vi "Set Print.vi"(8 "error in (no error)":errorcluster, 10 "On?":bool, 11 "MFC in":refnum<class "MFC.lvclass">) -> (0 "error out":errorcluster, 3 "MFC out":refnum<class "MFC.lvclass">)   [LabVIEW 2018, in "MFC Actor.lvlib" / "MFC.lvclass"]
uses:
  MFC.lvclass
  C:/Program Files/National Instruments/LabVIEW 2018/vi.lib/ActorFramework/Actor/Actor.lvclass
  <vilib>/ActorFramework/Actor/Actor.lvclass/Actor.ctl
  <vilib>/ActorFramework/Message Enqueuer/Message Enqueuer.lvclass/Message Enqueuer.ctl
  MFC.lvclass/MFC.ctl
  MFC Messages/Change Setpoint Msg/Change Setpoint Msg.lvclass/Change Setpoint Msg.ctl
  <vilib>/ActorFramework/Message Enqueuer/Init from Existing Queue.vi
  <vilib>/ActorFramework/Message Enqueuer/Enqueue.vi
  MFC Messages/Change Setpoint Msg/Change Setpoint Msg.lvclass
  C:/Program Files/National Instruments/LabVIEW 2018/vi.lib/ActorFramework/Message/Message.lvclass
  <vilib>/ActorFramework/Message Priority Queue/Priority Enqueue.vi
  <vilib>/ActorFramework/Message Enqueuer/Message Enqueuer.lvclass
  <vilib>/ActorFramework/Actor/Actor.lvclass
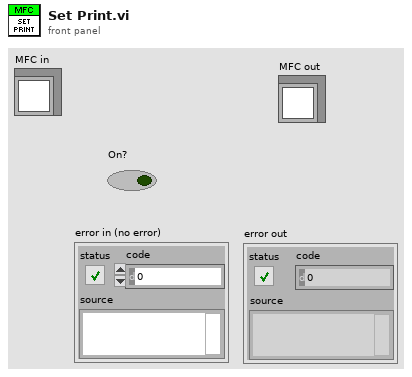
[diagram p1: front panel]
types:
  T1 = enum8{"Enabled", "Disabled", "Disabled and Grayed Out"}
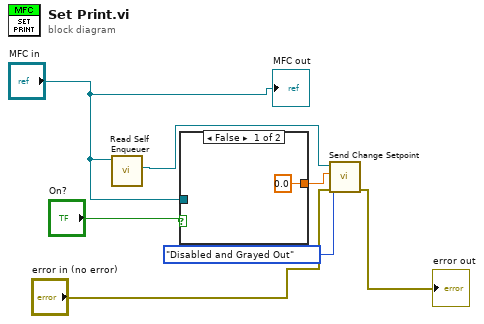
[diagram p0: block diagram]
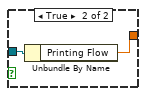
[diagram p2: hidden frame]
diagram:
  n1 = call <vilib>:"Read Self Enqueuer.vi"("Actor"="MFC in") -> ("Self Enqueuer"=w6:refnum<class "Message Enqueuer.lvclass">)  [unwired: 10 in]
  n2 = case shown="False" "On?" {
    tunnel: "MFC in" -> [_ w10]
    tunnel: [0.0 ("Printing Flow") w9] -> w5
    frame False {
    }
    frame True {
      n3 = Unbundle By Name(w10) -> ("Printing Flow"=w9:dbl)
    }
  }
  n4 = call "Send Change Setpoint.vi"("error in (no error)"="error in (no error)", "Disabled"=T1."Disabled and Grayed Out", "Setpoint"=w5, "Message Enqueuer in"=w6) -> ("error out"=→"error out":errorcluster)  [unwired: 6 in, 1 out]
  "MFC out" <- "MFC in"
